vi "Add Picture to VI Icon.vi"(8 "error in (no error)":errorcluster, 9 "Layer Name":string, 10 "Picture":picture, 11 "VI Reference":refnum<vi>) -> (0 "error out":errorcluster)   [LabVIEW 2012]
doc: "Adds a <b>Picture</b> as a separate user layer named <b>Layer Name</b> to the icon of the VI specified by <b>VI Reference</b>."
uses:
  <vilib>/LabVIEW Icon API/lv_icon/Classes/Layer/Layer.lvclass
  <vilib>/LabVIEW Icon API/lv_icon/Controls/LayerType.ctl
  <vilib>/LabVIEW Icon API/lv_icon/Classes/Icon/Icon.lvclass
  <vilib>/LabVIEW Icon API/LabVIEW Icon API.lvlib
panel:
  out "Updated Icon":picture
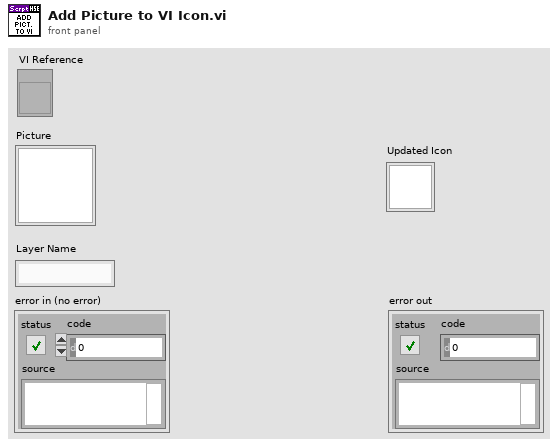
[diagram p1: front panel]
types:
  T1 = typedef "LayerType.ctl" = enum16{"Graphic", "Text", "Tool", "Graphic Drop"}
  T2 = typedef "imagedata.ctl" = cluster{"image type":i32, "image depth":i32, "image":u8[], "mask":u8[], "colors":u32[], "Rectangle":cluster{"left":i16, "top":i16, "right":i16, "bottom":i16}}
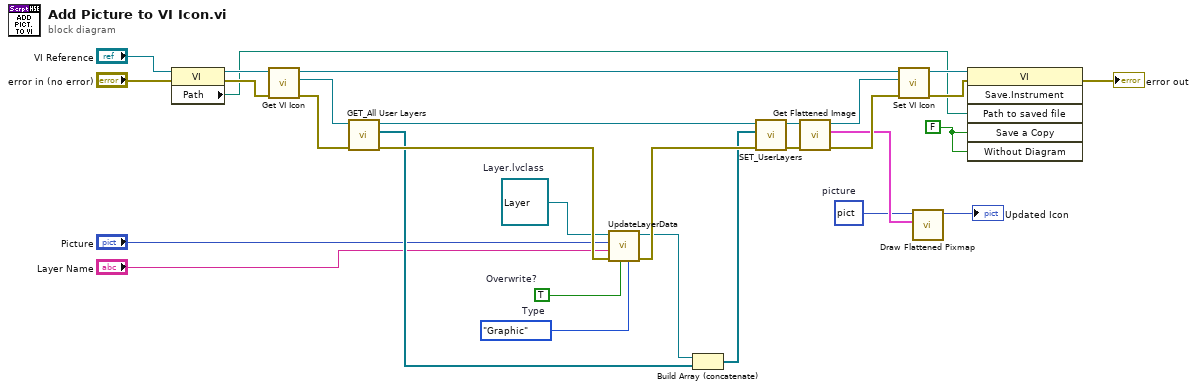
[diagram p0: block diagram]
diagram:
  w4 = FALSE ("Save a Copy")
  w12 = LayerType."Graphic"  # Type
  w13 = TRUE  # Overwrite?
  w16 = refnum<class "Layer.lvclass"> refnum  # Layer.lvclass
  w23 = picture data[5B]  # picture
  n1 = property class="VI"(reference="VI Reference", error in="error in (no error)") -> (reference out=w7:refnum<vi>, error out=w6:errorcluster, "Path"=w5:path)
  n2 = call <vilib>:"Get VI Icon.vi"("error in (no error)"=w6, "VI Refnum in"=w7) -> ("error out"=w17:errorcluster, "Icon"=w10:refnum<class "Icon.lvclass">, "VI Refnum out"=w27:refnum<vi>)  [unwired: 7 in]
  n3 = call-dynamic "GET_All User Layers.vi"("error in (no error)"=w17, "Icon.lvclass in"=w10) -> ("error out"=w30:errorcluster, "User Layer"=w14:refnum<class "Layer.lvclass">[], "Icon.lvclass out"=w20:refnum<class "Icon.lvclass">)  [unwired: 7 in]
  n4 = call <vilib>:"UpdateLayerData.vi"("Type"=w12, "Overwrite?"=w13, "error in"=w30, "LayerName"="Layer Name", "new picture"="Picture", "Active Layer"=w16) -> ("error out"=w29:errorcluster, "Layer.lvclass out"=w15:refnum<class "Layer.lvclass">)  [unwired: 4 in]
  n5 = Build Array (concatenate)(w15, w14) -> (w21:refnum<class "Layer.lvclass">[])
  n6 = call-dynamic "SET_UserLayers.vi"("error in (no error)"=w29, "Layers"=w21, "Icon.lvclass in"=w20) -> ("error out"=w18:errorcluster, "Icon.lvclass out"=w19:refnum<class "Icon.lvclass">)  [unwired: 7 in]
  n7 = call <vilib>:"Get Flattened Image.vi"("error in (no error)"=w18, "lv_icon.lvlib:Icon.lvclass in"=w19) -> ("error out"=w26:errorcluster, "Color Image"=w25:T2, "lv_icon.lvlib:Icon.lvclass out"=w22:refnum<class "Icon.lvclass">)  [unwired: 6 in, 1 out]
  n8 = call <vilib>:"Set VI Icon.vi"("error in (no error)"=w26, "Icon"=w22, "VI Refnum in"=w27) -> ("error out"=w8:errorcluster, "VI Refnum out"=w9:refnum<vi>)  [unwired: 7 in]
  n9 = call <vilib>:"Draw Flattened Pixmap.vi"("image data"=w25, "picture"=w23) -> ("new picture"=→"Updated Icon":picture)  [unwired: 7 in]
  n10 = invoke class="VI" method="Save.Instrument"(reference=w9, error in=w8, "Path to saved file"=w5, "Save a Copy"=w4, "Without Diagram"=w4) -> (error out=→"error out":errorcluster)  [unwired: 1 in, 5 out]
